vi "GetTestInformaton.vi"(8 "error in (no error)":errorcluster caption="错误输入（无错误）") -> (0 "error out":errorcluster caption="错误输出", 2 "SetTestInformaton":string[](array[string]), 3 "路径 2":path)   [LabVIEW 2018]
uses:
  Global.vi
  <vilib>/Utility/config.llb/Read Key (String).vi
  <vilib>/Utility/config.llb/NI_LVConfig.lvlib
panel:
  in  "路径":path
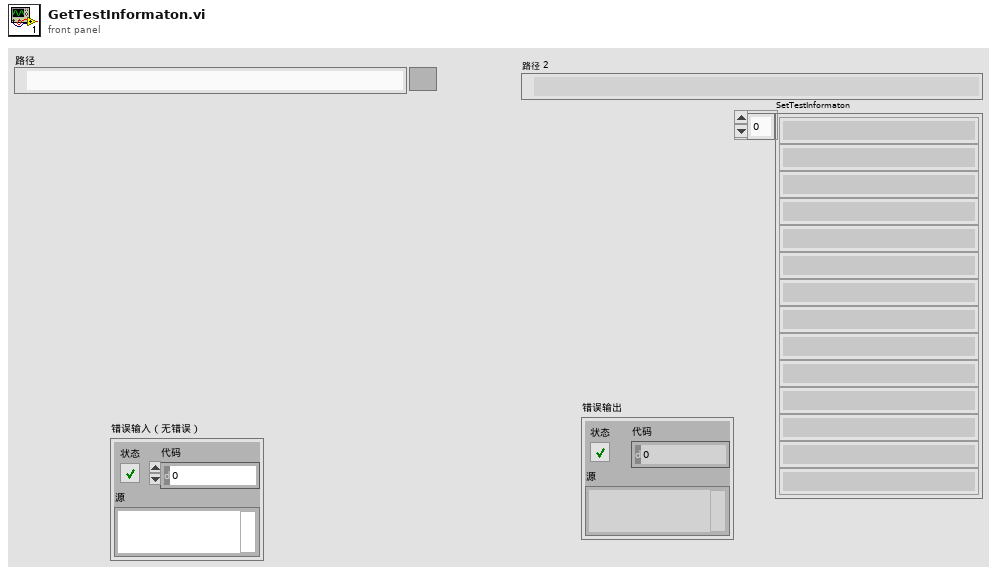
[diagram p1: front panel]
types:
  T1 = typedef "NI_LVConfig.lvlib/Config Data RefNum.ctl" = refnum<k1>
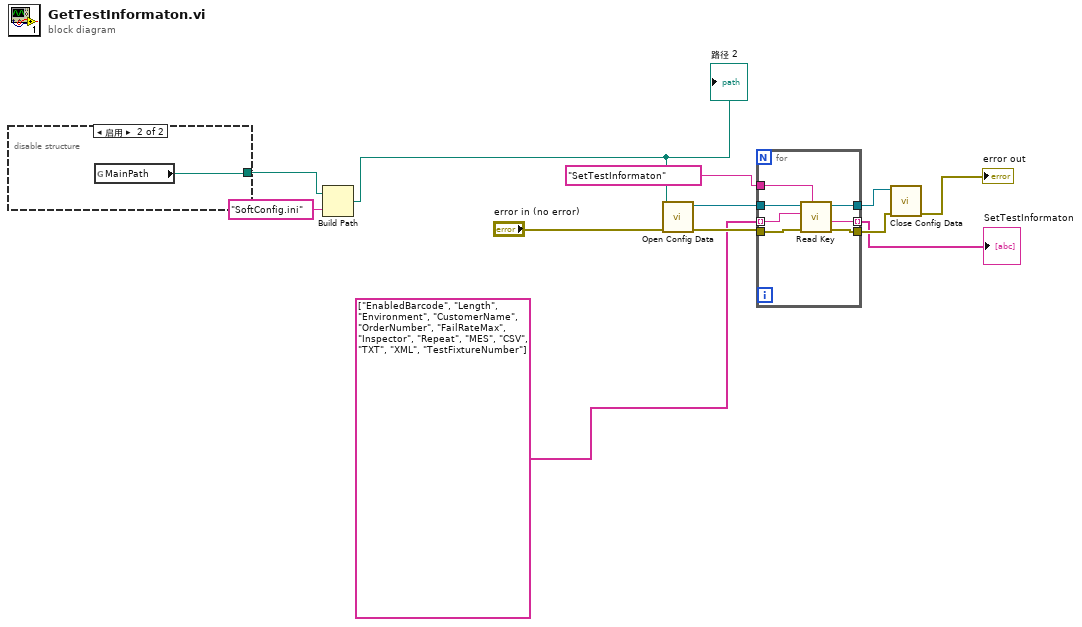
[diagram p0: block diagram]
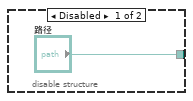
[diagram p2: hidden frame]
diagram:
  n1 = disable-structure shown="启用" {
    disable-tunnel: ["路径" w14] -> w6
    frame Disabled {
    }
    frame Enabled {
      n2 = global read "Global.vi" "MainPath"() -> (w14:path)
    }
  }
  n3 = Build Path(base path=w6, name or relative path="SoftConfig.ini" ("名称或相对路径")) -> (appended path=w4:path)
  "路径 2" <- w4
  n4 = call <vilib>:"Open Config Data.vi"("error in (no error)"="error in (no error)", "configuration file path"=w4) -> ("error out"=w2:errorcluster, "refnum"=w3:T1)  [unwired: 7 in, 1 out]
  n5 = for {
    tunnel: string[] ["EnabledBarcode", "Length", "Environment", "CustomerName", "OrderNumber", "FailRateMax", "Inspector", "Repeat", "MES", "CSV", "TXT", "XML", "TestFixtureNumber"] -> [w20] mode=indexing
    tunnel: w3 -> [w21]
    tunnel: [w19] -> w7 mode=indexing
    tunnel: [w18] -> w8
    tunnel: "SetTestInformaton" ("section") -> [w17]
    tunnel: [w16] -> w10
    tunnel: w2 -> [w15]
    n6 = call-poly <vilib>:"Read Key.vi"("section"=w17, "error in (no error)"=w15, "key"=w20, "refnum"=w21) -> ("error out"=w16:errorcluster, "value"=w19:string, "refnum out"=w18:T1)  [unwired: 4 in, 1 out]
  }
  "SetTestInformaton" <- w7
  n7 = call <vilib>:"Close Config Data.vi"("error in (no error)"=w10, "refnum"=w8) -> ("error out"=→"error out":errorcluster)  [unwired: 8 in, 1 out]
